vi "FormCommand2.vi"(1 "Parameters":string[](array[string]), 2 "Command":string) -> (0 "Command string":string)   [LabVIEW 2015]
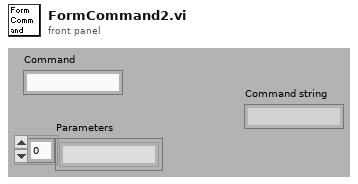
[diagram p1: front panel]
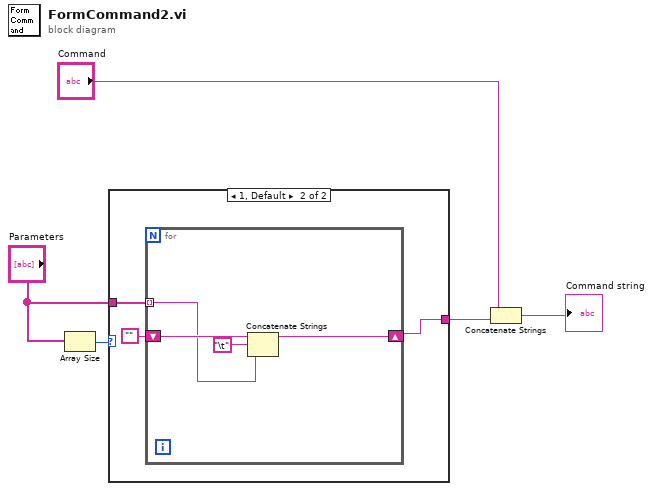
[diagram p0: block diagram]
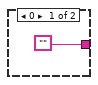
[diagram p2: hidden frame]
diagram:
  n1 = Array Size(array="Parameters") -> (size(s)=w4:i32)
  n2 = case shown="1, Default" w4 {
    tunnel: ["" w7] -> w3
    tunnel: "Parameters" -> [_ w9]
    frame 0 {
    }
    frame 1, Default {
      n3 = for {
        tunnel: w9 -> [w11] mode=indexing
        shift-right: [w10] -> w7
        shift-left: "" -> [w13]
        n4 = Concatenate Strings(w13, "\t", w11) -> (w10:string)
      }
    }
  }
  n5 = Concatenate Strings("Command", w3) -> (→"Command string":string)
